vi "ClientSrv Download.vi"(0 "file manipulation":T1, 5 "remote file":path, 9 "local file":path, 11 "error in (no error)":errorcluster, 12 "overwrite (F)":bool) -> (15 "error out":errorcluster)   [LabVIEW 2012]
doc: "Downloads a file from the server to the client. To limit memory usage, the download is performed in chunks. The duty cycle is throttled to 50% so as to not overtax the server."
uses:
  served/ClientSrv Server File Manipulation_srv.ctl
  typedefs/t_ClientSrv Server File Manipulation Methods.ctl
  typedefs/t_ClientSrv Access Levels.ctl
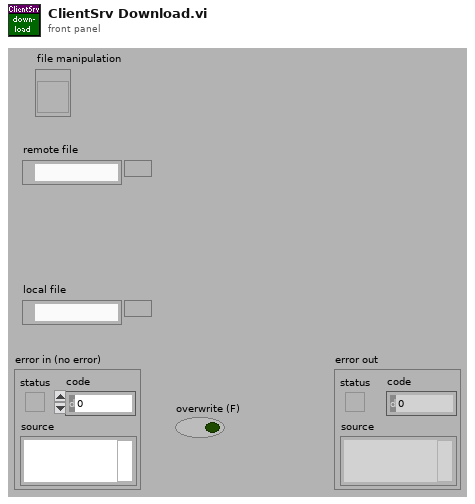
[diagram p1: front panel]
types:
  T1 = typedef "ClientSrv Server File Manipulation_srv.ctl" = refnum<vi>
  T2 = typedef "t_ClientSrv Access Levels.ctl" = enum16{"observer", "operator", "local"}
  T3 = typedef "t_ClientSrv Server File Manipulation Methods.ctl" = enum16{"close", "list", "open", "new", "read", "write", "newdir", "info", "rename", "delete"}
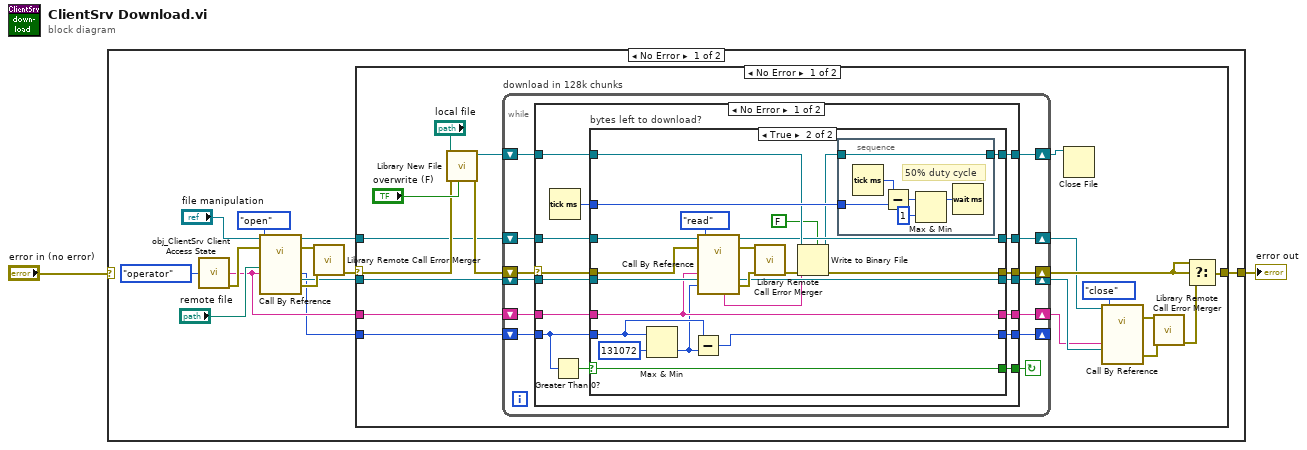
[diagram p0: block diagram]
diagram:
  n1 = case shown="No Error" "error in (no error)" {
    selector: "error in (no error)" -> [_ w105]
    tunnel: [w6 w105] -> w2
    frame No Error {
      n2 = call "obj_ClientSrv Client Access State.vi"("access level (observer)"=t_ClientSrv_Access_Levels."operator") -> ("certificate"=w5:string, "error out"=w14:errorcluster)  [unwired: 13 in]
      n3 = call-by-ref "?"(reference="file manipulation", error in=w14, "method"=t_ClientSrv_Server_File_Manipulation_Methods."open", "path"="remote file", "certificate"=w5) -> (reference out=w7:T1, error out=w11:errorcluster, "length"=w4:i32, "refnum out"=w8:refnum<file>, 15:"error out"=w10:errorcluster)  [unwired: 5 in, 5 out]
      n4 = call "Library Remote Call Error Merger.vi"("call by reference node error"=w11, "called VI error (no error)"=w10) -> ("error out"=w9:errorcluster)  [unwired: 13 in]
      n5 = case shown="No Error" w9 {
        selector: w9 -> [w18 w104]
        tunnel: w8 -> [w17 _]
        tunnel: w4 -> [w34 _]
        tunnel: w7 -> [w16 _]
        tunnel: [w26 w104] -> w6
        tunnel: w5 -> [w33 _]
        frame No Error {
          n6 = call "Library New File.vi"("overwrite (F)"="overwrite (F)", "error in (no error)"=w18, "file path"="local file") -> ("error out"=w19:errorcluster, "refnum"=w20:refnum<file>)  [unwired: 7 in]
          n7 = while "download in 128k chunks" {
            shift-right: [w43] -> w23
            shift-left: w20 -> [w44]
            shift-right: [w40] -> _
            shift-left: w34 -> [w47]
            shift-right: [w38] -> w25
            shift-left: w16 -> [w39]
            shift-right: [w36] -> w31
            shift-left: w17 -> [w37]
            shift-right: [w45] -> w28
            shift-left: w19 -> [w46]
            shift-right: [w35] -> w24
            shift-left: w33 -> [w41]
            stop <- w42 continue-if-true
            n8 = case shown="No Error" w46 {
              selector: w46 -> [w56 w103]
              tunnel: w47 -> [w59 w101]
              tunnel: [w52 w103] -> w45
              tunnel: [w53 w102] -> w43
              tunnel: w44 -> [w57 w102]
              tunnel: [w61 _] -> w42
              tunnel: w41 -> [w60 w98]
              tunnel: [w58 w101] -> w40
              tunnel: w39 -> [w55 w100]
              tunnel: [w54 w100] -> w38
              tunnel: w37 -> [w50 w99]
              tunnel: [w49 w99] -> w36
              tunnel: [w48 w98] -> w35
              frame No Error {
                n9 = Tick Count (ms)() -> (millisecond timer value=w51:u32)
                n10 = Greater Than 0?(x=w59) -> (x > 0?=w62:bool)
                n11 = case "bytes left to download?" shown="True" w62 {
                  selector: w62 -> [w69 w91]
                  tunnel: [w69 w91] -> w61
                  tunnel: w60 -> [w63 w80]
                  tunnel: w59 -> [w68 w89]
                  tunnel: [w68 w88] -> w58
                  tunnel: w57 -> [w66 w76]
                  tunnel: w56 -> [w65 w79]
                  tunnel: w55 -> [w67 w87]
                  tunnel: [w67 w75] -> w54
                  tunnel: [w66 w74] -> w53
                  tunnel: [w65 w77] -> w52
                  tunnel: w51 -> [_ w83]
                  tunnel: w50 -> [w64 w82]
                  tunnel: [w64 w81] -> w49
                  tunnel: [w63 w80] -> w48
                  frame False {
                  }
                  frame True {
                    n12 = Max & Min(x=w89, y=131072) -> (min(x,y)=w78:i32)  [unwired: 1 out]
                    n13 = Subtract(x=w89, y=w78) -> (x-y=w88:i32)
                    n14 = call-by-ref "?"(reference=w87, error in=w79, "method"=t_ClientSrv_Server_File_Manipulation_Methods."read", "certificate"=w80, "refnum in"=w82, "read amount"=w78) -> (reference out=w75:T1, error out=w85:errorcluster, "refnum out"=w81:refnum<file>, "data out"=w71:string, 15:"error out"=w84:errorcluster)  [unwired: 4 in, 5 out]
                    n15 = call "Library Remote Call Error Merger.vi"("call by reference node error"=w85, "called VI error (no error)"=w84) -> ("error out"=w72:errorcluster)  [unwired: 13 in]
                    n16 = Write to Binary File(file (use dialog)=w76, data=w71, error in=w72, 5:FALSE ("prepend array or string size? (T)")) -> (refnum out=w73:refnum<file>, error out=w77:errorcluster)  [unwired: 2 in, 1 out]
                    n17 = stacked-sequence {
                      tunnel: w83 -> [w97]
                      tunnel: w73 -> [w92]
                      tunnel: [w92] -> w74
                      frame #0 {
                        # "50% duty cycle"
                        n18 = Tick Count (ms)() -> (millisecond timer value=w96:u32)
                        n19 = Subtract(x=w96, y=w97) -> (x-y=w95:u32)
                        n20 = Max & Min(x=w95, y=u32 1) -> (max(x,y)=w93:u32)  [unwired: 1 out]
                        n21 = Wait (ms)(milliseconds to wait=w93) -> ()  [unwired: 1 out]
                      }
                    }
                  }
                }
              }
              frame Error {
              }
            }
          }
          n22 = Close File(refnum=w23) -> ()  [unwired: 1 in, 2 out]
          n23 = call-by-ref "?"(reference=w25, "method"=t_ClientSrv_Server_File_Manipulation_Methods."close", "certificate"=w24, "refnum in"=w31) -> (error out=w30:errorcluster, 15:"error out"=w29:errorcluster)  [unwired: 6 in, 8 out]
          n24 = call "Library Remote Call Error Merger.vi"("call by reference node error"=w30, "called VI error (no error)"=w29) -> ("error out"=w27:errorcluster)  [unwired: 13 in]
          n25 = Select(t=w28, s=w28, f=w27) -> (s? t:f=w26:errorcluster)
        }
        frame Error {
        }
      }
    }
    frame Error {
    }
  }
  "error out" <- w2
